vi "MDAQ_KeepTime.vi"(7 "Delta T (s)":dbl, 8 "State in":T3, 9 "Cluster In":T1 {"CV"."Temperature Array" scale=0.0..100.0}, 11 "Slide in":refnum<vi>) -> (0 "State Out":T3, 1 "Cluster Out":T1 {"CV"."Temperature Array" scale=0.0..100.0}, 3 "Progress":u8, 4 "Elapsed Out":dbl)   [LabVIEW 2021]
uses:
  Status_Def.ctl
  GUI_Def.ctl
  Mode_Enum.ctl
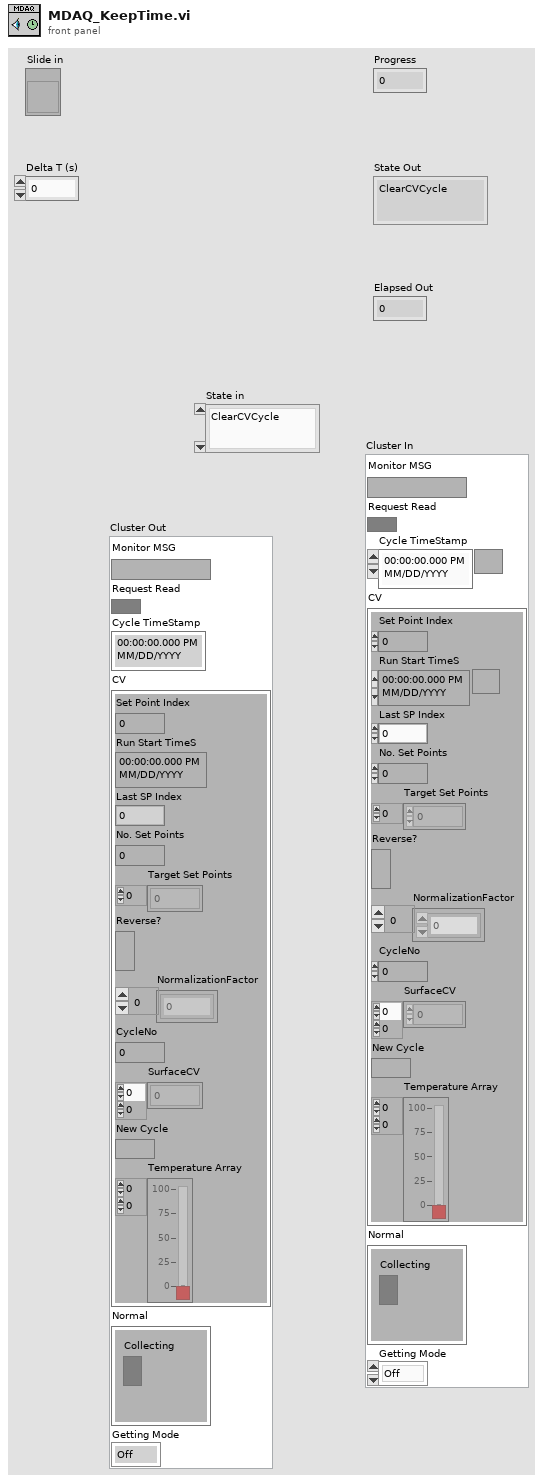
[diagram p1: front panel]
types:
  T1 = typedef "GUI_Def.ctl" = cluster{"Monitor MSG":string, "Request Read":bool, "Cycle TimeStamp":timestamp, "CV":cluster{"Set Point Index":u32, "Run Start TimeS":timestamp, "Last SP Index":u32, "No. Set Points":u32, "Target Set Points":i32[], "Reverse?":bool, "NormalizationFactor":i32[], "CycleNo":i32, "SurfaceCV":dbl[][], "New Cycle":bool, "Temperature Array":dbl[][]}, "Normal":cluster{"Collecting":bool}, "Getting Mode":T2}
  T2 = typedef "Mode_Enum.ctl" = enum16{"Off", "Normal", "CV+Temp", "CV"}
  T3 = typedef "Status_Def.ctl" = enum16{"ClearCVCycle", "WriteCVData", "SendRamp", "LoadSpectrum", "RefreshCV", "SaveCVPlot", "GetCVSpectrum", "ConfigCV", "StopCV", "StartCV", "SaveSpectrum", "Clear Spectrum", "StopCollecting", "StopAq", "StartAq", "Reset MDAQ", "Get Spectrum", "Clear Monitor", "Idle", "String Send", "Settings Send", "Read Help"}
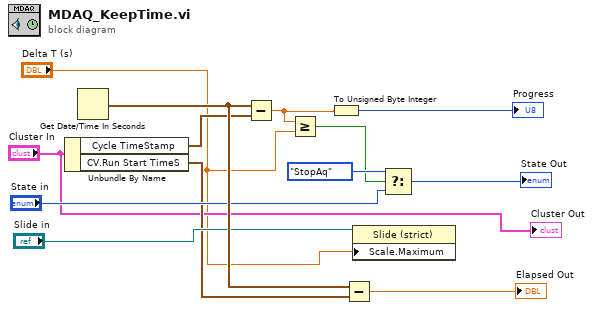
[diagram p0: block diagram]
diagram:
  n1 = Unbundle By Name("Cluster In") -> ("Cycle TimeStamp"=w3:timestamp, "CV.Run Start TimeS"=w4:timestamp)
  n2 = Get Date/Time In Seconds() -> (seconds since 1Jan1904=w11:timestamp)
  n3 = Subtract(x=w11, y=w3) -> (x-y=w9:dbl)
  n4 = Greater Or Equal?(x=w9, y="Delta T (s)") -> (x >= y?=w5:bool)
  n5 = To Unsigned Byte Integer(number=w9) -> (unsigned 8bit integer=→"Progress":u8)
  n6 = Subtract(x=w11, y=w4) -> (x-y=→"Elapsed Out":dbl)
  n7 = property class="Slide (strict)"(reference="Slide in", "Scale.Maximum"="Delta T (s)") -> ()  [unwired: 1 in, 2 out]
  n8 = Select(t=Status_Def."StopAq", s=w5, f="State in") -> (s? t:f=→"State Out":T3)
  "Cluster Out" <- "Cluster In"
